vi "Map Microcontroller Memory.vi"(0 ".hex lines":T1(array[cluster]), 2 "Memory Max. Size":i32=524288, 5 "Memory Address":u32[](array[numeric]), 7 "It's a Data Record Type":bool[](array[boolean]), 11 "error in":errorcluster) -> (4 "Complete Memory Map (512KBytes)":i16[](array[numeric]), 15 "error out":errorcluster)   [LabVIEW 2010]
panel:
  out "Occupied Memory":i32[](graph)=[86944, 113022, 115380, 131232, 127708, 129132, 127717, 119274, 119924, 121775, 124335, 114307, 119076, 67258, -1024, -1024, -1024, -1024, -1024, -1024, -1024, -1024, -1024, -1024, -1024, -1024, -1024, -1024, -1024, -1024, -1024, -1024, -1024, -1024, -1024, -1024, -1024, -1024, -1024, -1024, -1024, -1024, -1024, -1024, -1024, -1024, -1024, -1024, -1024, -1024, -1024, -1024, -1024, -1024, -1024, -1024, -1024, -1024, -1024, -1024, -1024, -1024, -1024, -1024, -1024, -1024, -1024, -1024, -1024, -1024, -1024, -1024, -1024, -1024, -1024, -1024, -1024, -1024, -1024, -1024, -1024, -1024, -1024, -1024, -1024, -1024, -1024, -1024, -1024, -1024, -1024, -1024, -1024, -1024, -1024, -1024, -1024, -1024, -1024, -1024, -1024, -1024, -1024, -1024, -1024, -1024, -1024, -1024, -1024, -1024, -1024, -1024, -1024, -1024, -1024, -1024, -1024, -1024, -1024, -1024, -1024, -1024, -1024, -1024, -1024, -1024, -1024, -1024, -1024, -1024, -1024, -1024, -1024, -1024, -1024, -1024, -1024, -1024, -1024, -1024, -1024, -1024, -1024, -1024, -1024, -1024, -1024, -1024, -1024, -1024, -1024, -1024, -1024, -1024, -1024, -1024, -1024, -1024, -1024, -1024, -1024, -1024, -1024, -1024, -1024, -1024, -1024, -1024, -1024, -1024, -1024, -1024, -1024, -1024, -1024, -1024, -1024, -1024, -1024, -1024, -1024, -1024, -1024, -1024, -1024, -1024, -1024, -1024, -1024, -1024, -1024, -1024, -1024, -1024, -1024, -1024, -1024, -1024, -1024, -1024, -1024, -1024, -1024, -1024, -1024, -1024, -1024, -1024, -1024, -1024, -1024, -1024, -1024, -1024, -1024, -1024, -1024, -1024, -1024, -1024, -1024, -1024, -1024, -1024, -1024, -1024, -1024, -1024, -1024, -1024, -1024, -1024, -1024, -1024, -1024, -1024, -1024, -1024, -1024, -1024, -1024, -1024, -1024, -1024, -1024, -1024, -1024, -1024, -1024, -1024, -1024, -1024, -1024, -1024, -1024, -1024, -1024, -1024, -1024, -1024, -1024, -1024, -1024, -1024, -1024, -1024, -1024, -1024, -1024, -1024, -1024, -1024, -1024, -1024, -1024, -1024, -1024, -1024, -1024, -1024, -1024, -1024, -1024, -1024, -1024, -1024, -1024, -1024, -1024, -1024, -1024, -1024, -1024, -1024, -1024, -1024, -1024, -1024, -1024, -1024, -1024, -1024, -1024, -1024, -1024, -1024, -1024, -1024, -1024, -1024, -1024, -1024, -1024, -1024, -1024, -1024, -1024, -1024, -1024, -1024, -1024, -1024, -1024, -1024, -1024, -1024, -1024, -1024, -1024, -1024, -1024, -1024, -1024, -1024, -1024, -1024, -1024, -1024, -1024, -1024, -1024, -1024, -1024, -1024, -1024, -1024, -1024, -1024, -1024, -1024, -1024, -1024, -1024, -1024, -1024, -1024, -1024, -1024, -1024, -1024, -1024, -1024, -1024, -1024, -1024, -1024, -1024, -1024, -1024, -1024, -1024, -1024, -1024, -1024, -1024, -1024, -1024, -1024, -1024, -1024, -1024, -1024, -1024, -1024, -1024, -1024, -1024, -1024, -1024, -1024, -1024, -1024, -1024, -1024, -1024, -1024, -1024, -1024, -1024, -1024, -1024, -1024, -1024, -1024, -1024, -1024, -1024, -1024, -1024, -1024, -1024, -1024, -1024, -1024, -1024, -1024, -1024, -1024, -1024, -1024, -1024, -1024, -1024, -1024, -1024, -1024, -1024, -1024, -1024, -1024, -1024, -1024, -1024, -1024, -1024, -1024, -1024, -1024, -1024, -1024, -1024, -1024, -1024, -1024, -1024, -1024, -1024, -1024, -1024, -1024, -1024, -1024, -1024, -1024, -1024, -1024, -1024, -1024, -1024, -1024, -1024, -1024, -1024, -1024, -1024, -1024, -1024, -1024, -1024, -1024, -1024, -1024, -1024, -1024, -1024, -1024, -1024, -1024, -1024, -1024, -1024, -1024, -1024, -1024, -1024, -1024, -1024, -1024, -1024, -1024, -1024, -1024, -1024, -1024, -1024, -1024, -1024, -1024, -1024, -1024, -1024, -1024, -1024, -1024, -1024, -1024, -1024, -1024, -1024, -1024, -1024, -1024]
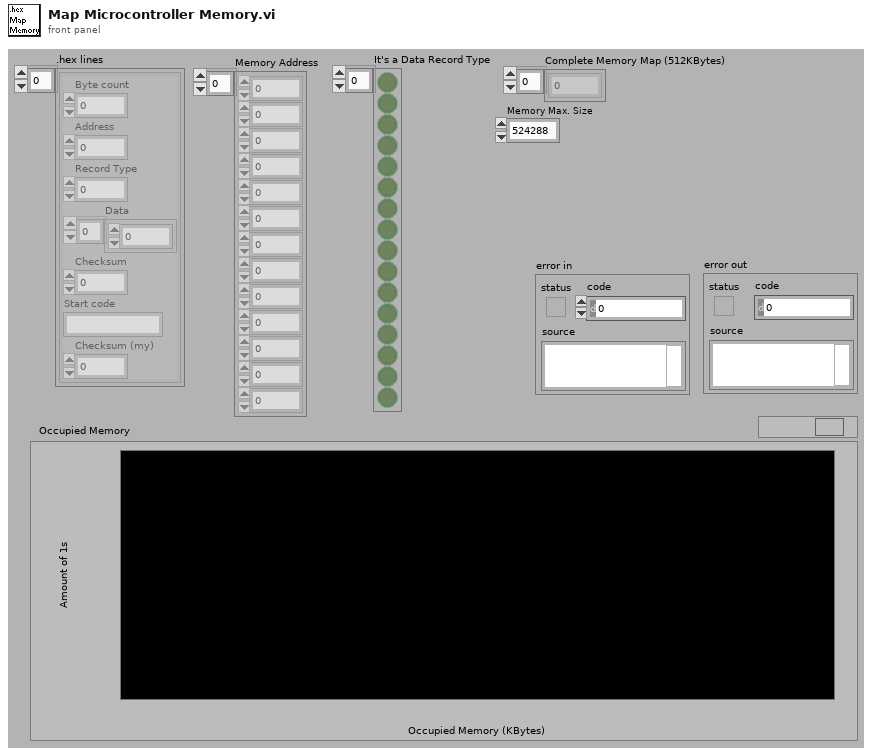
[diagram p1: front panel]
types:
  T1 = cluster{"Byte count":u8, "Address":u16, "Record Type":u8, "Data":u8[], "Checksum":u8, "Start code":string, "Checksum (my)":u8}[]
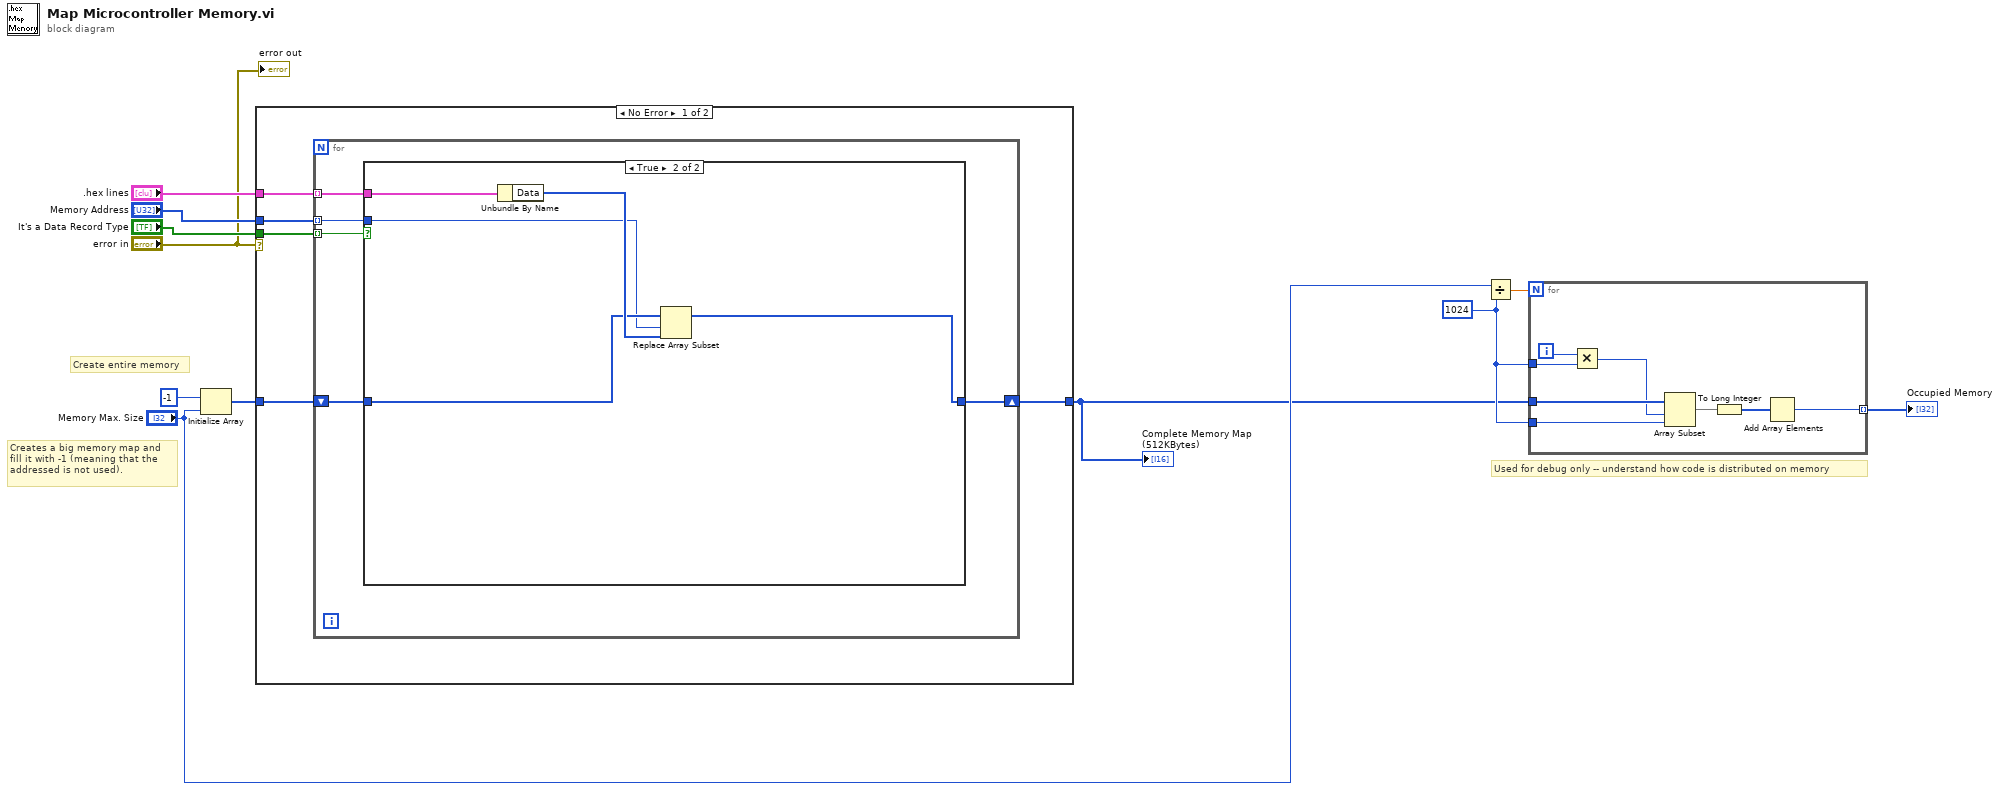
[diagram p0: block diagram]
diagram:
  w7 = 1024 ("y")
  # "Creates a big memory map and\nfill it with -1 (meaning that the\naddressed is not used)."
  # "Used for debug only -- understand how code is distributed on memory"
  # "Create entire memory"
  n1 = Initialize Array(i16 -1 ("element"), "Memory Max. Size") -> (w5:i16[])
  n2 = case shown="No Error" "error in" {
    tunnel: ".hex lines" -> [w16 _]
    tunnel: "Memory Address" -> [w15 _]
    tunnel: "It's a Data Record Type" -> [w14 _]
    tunnel: w5 -> [w13 w28]
    tunnel: [w12 w28] -> w1
    frame No Error {
      n3 = for {
        tunnel: w16 -> [w20] mode=indexing
        tunnel: w15 -> [w18] mode=indexing
        tunnel: w14 -> [w21] mode=indexing
        shift-right: [w17] -> w12
        shift-left: w13 -> [w19]
        n4 = case shown="True" w21 {
          tunnel: w20 -> [_ w27]
          tunnel: w19 -> [w22 w25]
          tunnel: w18 -> [_ w24]
          tunnel: [w22 w23] -> w17
          frame False {
          }
          frame True {
            n5 = Unbundle By Name(w27) -> ("Data"=w26:u8[])
            n6 = Replace Array Subset(array=w25, new element=w26, index=w24) -> (w23:i16[])
          }
        }
      }
    }
    frame Error {
    }
  }
  "Complete Memory Map (512KBytes)" <- w1
  n7 = Divide(x="Memory Max. Size", y=w7) -> (x/y=w6:dbl)
  n8 = for {
    N: w6 -> [_]
    tunnel: w1 -> [w36]
    tunnel: w7 -> [w34]
    tunnel: w7 -> [w32]
    tunnel: [w29] -> w8 mode=indexing
    i -> [w35]
    n9 = Multiply(x=w35, y=w34) -> (x*y=w33:i32)
    n10 = Array Subset(array=w36, index=w33, length=w32) -> (w31:i16[])
    n11 = To Long Integer(number=w31) -> (32bit integer=w30:i32[])
    n12 = Add Array Elements(numeric array=w30) -> (sum=w29:i32)
  }
  "Occupied Memory" <- w8
  "error out" <- "error in"
